vi "Insert Case Structure.vi"(0 "ITest Executive in":refnum<class "ITest Executive.lvclass">, 1 "Name":string, 2 "Unique ID":string, 3 "Insertion Index":i32=-1, 4 "Assertions":refnum<class "Assert.lvclass">[](array[class]), 5 "error in (no error)":errorcluster, 6 "Parent ID":string, 7 "X Variables":string[](array[string]), 9 "Y Variables":string[](array[string]), 11 "Conditional Branches":string[](array[string]), 13 "\"Else\" Conditional Branch":string) -> (12 "Unique ID out":string, 14 "ITest Executive out":refnum<class "ITest Executive.lvclass">, 17 "Replaced?":bool, 19 "error out":errorcluster)   [LabVIEW 2017, in "Test Executive.lvlib" / "ITest Executive.lvclass"]
uses:
  <vilib>/gpm_packages/@cs/test-executive/Source/Test Executive/ITestExecutive/ITest Executive.lvclass
  <vilib>/gpm_packages/@cs/run-time-assertions/Source/Assert/Assert.lvclass
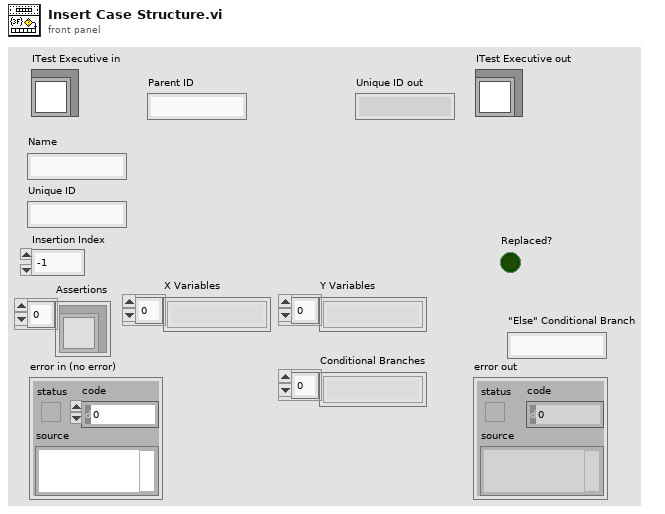
[diagram p1: front panel]
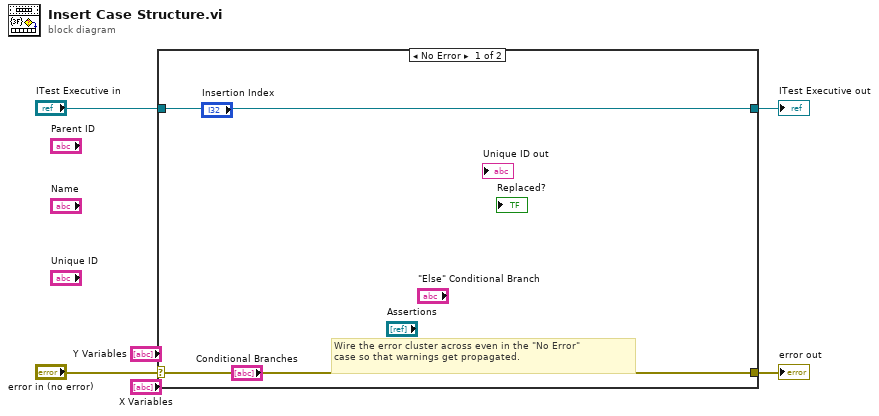
[diagram p0: block diagram]
diagram:
  n1 = case shown="No Error" "error in (no error)" {
    selector: "error in (no error)" -> [w5 w8]
    tunnel: [w5 w8] -> w3
    tunnel: [w6 w7] -> w1
    tunnel: "ITest Executive in" -> [w6 w7]
    frame No Error {
      # "Wire the error cluster across even in the \"No Error\"\ncase so that warnings get propagated."
    }
    frame Error {
    }
  }
  "error out" <- w3
  "ITest Executive out" <- w1
